vi "Create User Events.vi"(8 "Error In":errorcluster) -> (0 "Error Out":errorcluster, 1 "Event Refnum":refnum<event-registration>, 2 "Events":T1)   [LabVIEW 2011, in "LMH-Xbox-One-Controller.lvlib"]
uses:
  LMH-Xbox-One-Controller.lvlib
  Type Defs/Events.ctl
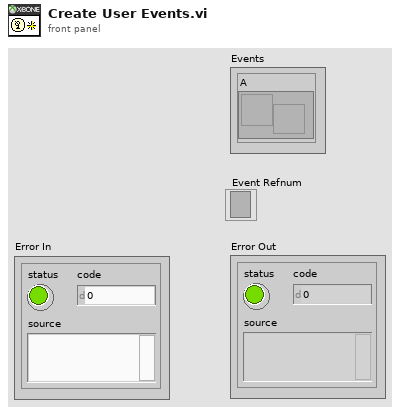
[diagram p1: front panel]
types:
  T1 = typedef "LMH-Xbox-One-Controller.lvlib/Events.ctl" = cluster{"A":refnum<user-event>, "B":refnum<user-event>, "X":refnum<user-event>, "Y":refnum<user-event>, "Left Bumper":refnum<user-event>, "Right Bumper":refnum<user-event>, "View":refnum<user-event>, "Menu":refnum<user-event>, "Left Stick":refnum<user-event>, "Right Stick":refnum<user-event>}
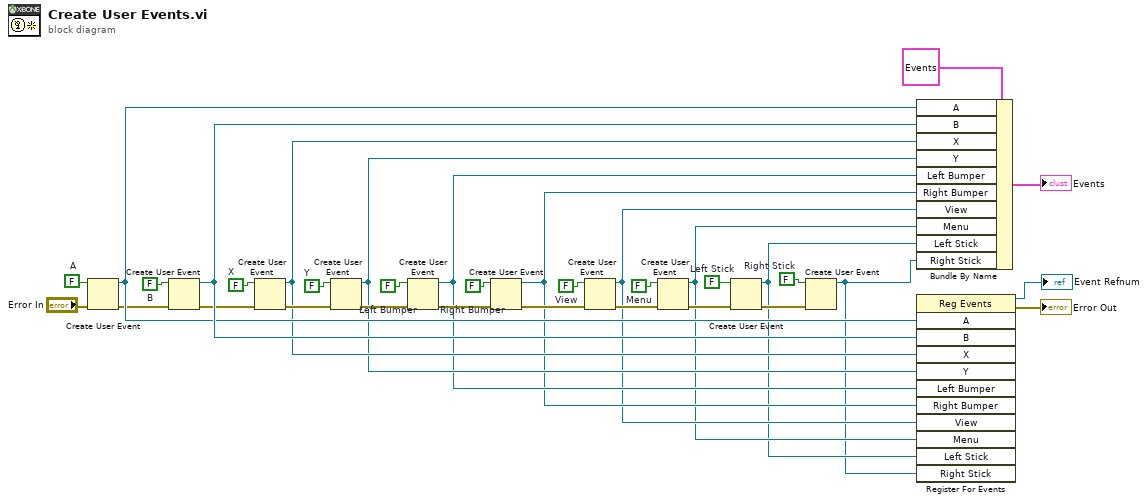
[diagram p0: block diagram]
diagram:
  w18 = FALSE  # Right Stick
  w19 = FALSE  # Left Stick
  w22 = FALSE  # Menu
  w23 = FALSE  # View
  w24 = FALSE  # Right Bumper
  w25 = FALSE  # Left Bumper
  w26 = FALSE  # Y
  w27 = FALSE  # X
  w29 = FALSE  # B
  w28 = FALSE  # A
  n1 = Create User Event(user event datatype=w28, error in="Error In") -> (user event=w33:refnum<user-event>, error out=w21:errorcluster)
  n2 = Create User Event(user event datatype=w29, error in=w21) -> (user event=w34:refnum<user-event>, error out=w20:errorcluster)
  n3 = Create User Event(user event datatype=w27, error in=w20) -> (user event=w10:refnum<user-event>, error out=w17:errorcluster)
  n4 = Create User Event(user event datatype=w26, error in=w17) -> (user event=w9:refnum<user-event>, error out=w16:errorcluster)
  n5 = Create User Event(user event datatype=w25, error in=w16) -> (user event=w8:refnum<user-event>, error out=w15:errorcluster)
  n6 = Create User Event(user event datatype=w24, error in=w15) -> (user event=w7:refnum<user-event>, error out=w14:errorcluster)
  n7 = Create User Event(user event datatype=w23, error in=w14) -> (user event=w6:refnum<user-event>, error out=w13:errorcluster)
  n8 = Create User Event(user event datatype=w22, error in=w13) -> (user event=w5:refnum<user-event>, error out=w12:errorcluster)
  n9 = Create User Event(user event datatype=w19, error in=w12) -> (user event=w4:refnum<user-event>, error out=w11:errorcluster)
  n10 = Create User Event(user event datatype=w18, error in=w11) -> (user event=w3:refnum<user-event>)  [unwired: 1 out]
  n11 = Bundle By Name(cluster=T1 {"A"=refnum, "B"=refnum, "X"=refnum, "Y"=refnum, "Left Bumper"=refnum, "Right Bumper"=refnum, "View"=refnum, "Menu"=refnum, "Left Stick"=refnum, "Right Stick"=refnum} ("Events"), "A"=w33, "B"=w34, "X"=w10, "Y"=w9, "Left Bumper"=w8, "Right Bumper"=w7, "View"=w6, "Menu"=w5, "Left Stick"=w4, "Right Stick"=w3) -> (→"Events":T1)
  n12 = register-events(w33, w34, w10, w9, w8, w7, w6, w5, w4, w3) -> (reference out=→"Event Refnum":refnum<event-registration>, error out=→"Error Out":errorcluster)  [unwired: 2 in]
